vi "글로별 변수 실습.vi"() -> ()   [LabVIEW 2020]
panel:
  out "배열":dbl[](array[numeric])
  in  "정지":bool
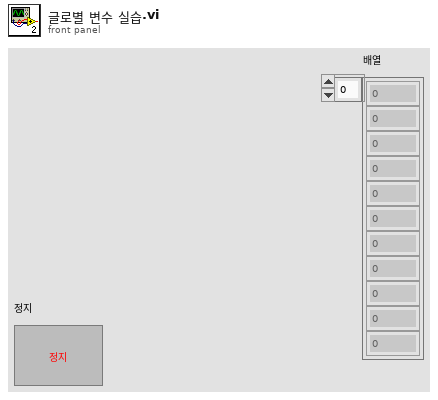
[diagram p1: front panel]
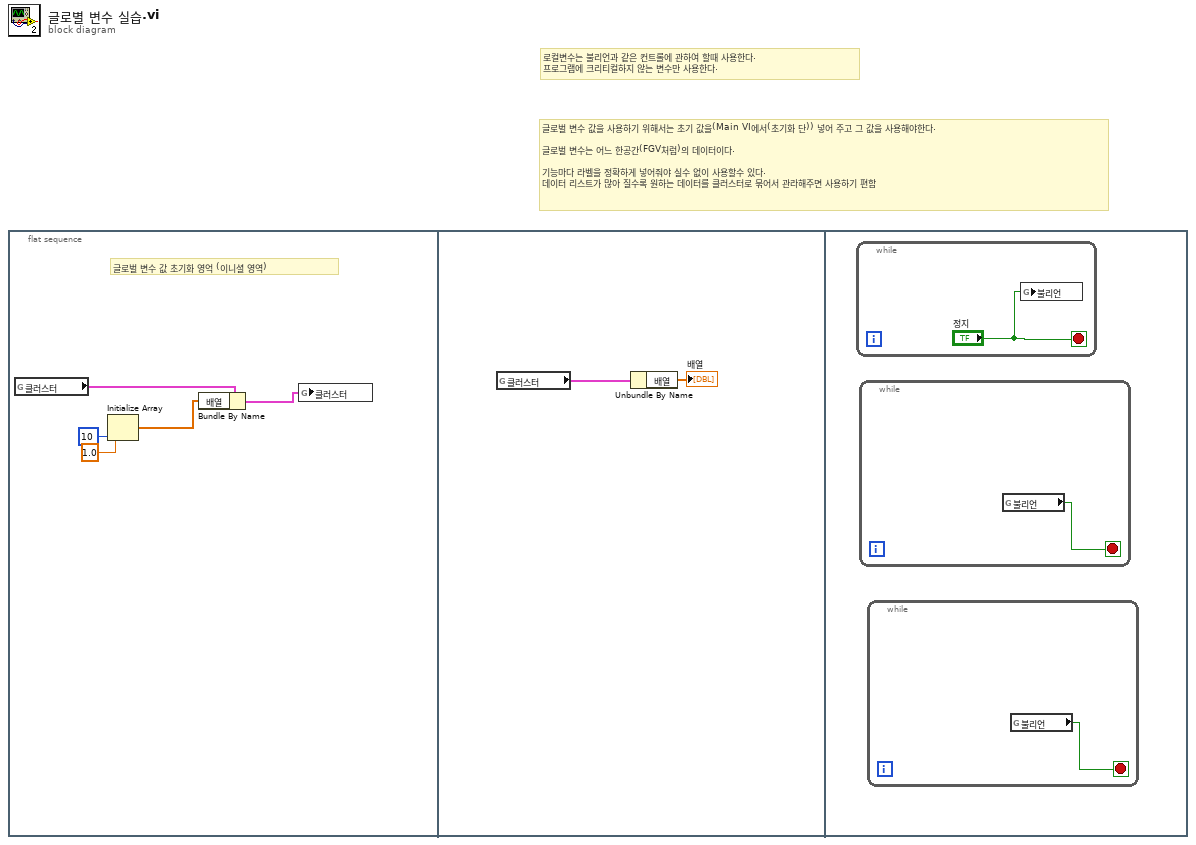
[diagram p0: block diagram]
diagram:
  # "로컬변수는 불리언과 같은 컨트롤에 관하여 할때 사용한다.\n프로그램에 크리티컬하지 않는 변수만 사용한다."
  # "글로벌 변수 값을 사용하기 위해서는 초기 값을(Main VI에서(초기화 단)) 넣어 주고 그 값을 사용해야한다.\n\n글로벌 변수는 어느 한공간(FGV처럼)의 데이터이다.\n\n기능마다 라벨을 정확하게 넣어줘야 실수 없이 사용할수 있다.\n데이터 리스트가 많아 질수록 원하는 데이터를 클러스터로 묶어서 관라해주면 사용하기 편함"
  n1 = flat-sequence {
    frame #0 {
      # "글로벌 변수 값 초기화 영억 (이니셜 영역)"
      n2 = global read "글로벌 2.vi" "클러스터"() -> (w5:cluster{"배열":dbl[], "불리언":bool})
      n3 = Initialize Array(1.0 ("원소"), 10 ("차원 크기")) -> (w2:dbl[])
      n4 = Bundle By Name(cluster=w5, "배열"=w2) -> (w1:cluster{"배열":dbl[], "불리언":bool})
      n5 = global write "글로벌 2.vi" "클러스터"(w1) -> ()
    }
    frame #1 {
      n6 = global read "글로벌 2.vi" "클러스터"() -> (w7:cluster{"배열":dbl[], "불리언":bool})
      n7 = Unbundle By Name(w7) -> ("배열"=→"배열":dbl[])
    }
    frame #2 {
      n8 = while {
        stop <- "정지" stop-if-true
        n9 = global write "글로벌 2.vi" "불리언"("정지") -> ()
      }
      n10 = while {
        stop <- w9 stop-if-true
        n11 = global read "글로벌 2.vi" "불리언"() -> (w9:bool)
      }
      n12 = while {
        stop <- w8 stop-if-true
        n13 = global read "글로벌 2.vi" "불리언"() -> (w8:bool)
      }
    }
  }
